vi "test Filters.vi"(8 "error in (no error)":errorcluster, 11 "BM Filters in":refnum<class "BM Filters.lvclass">) -> (0 "error out":errorcluster, 3 "BM Filters out":refnum<class "BM Filters.lvclass">)   [LabVIEW 2016, in "BM Filters.lvclass"]
uses:
  BM Filters.lvclass
  Filters/Filter/Filter.lvclass
  Frames & Messages/TypeDefs/Command Type.ctl
  BCI-1553 API.lvlib
  Filters/TypeDefs/Filter Configuration.ctl
  1553 Component/1553 Component.lvclass
  Bus Monitor/TypeDefs/Bus Monitor Configuration.ctl
  Bus Monitor/Bus Monitor.lvclass
  1553 Board/1553 Board.lvclass
  PPLs/FPGA Interface.lvlibp/FPGA Interface/FPGA Interface.lvclass
  Utilities/FPGA Interface/FPGA Interface.lvclass
  D:/SVN/Products/BCI-1553/Software/Development/2016/RealTime/1553 SubComponent/1553 SubComponent.lvclass
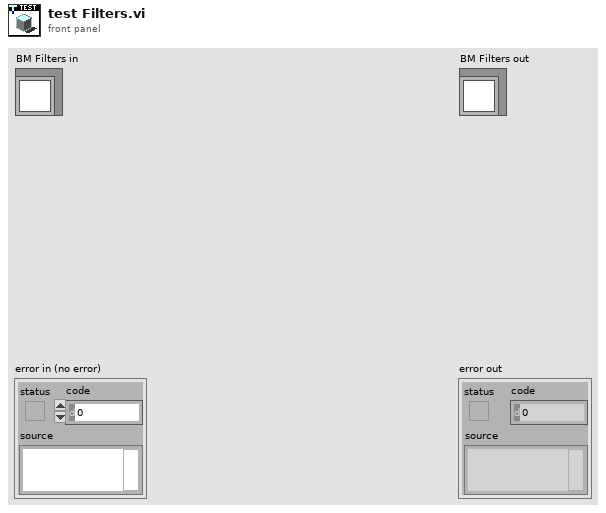
[diagram p1: front panel]
types:
  T1 = typedef "BCI-1553 API.lvlib/Bus Monitor.lvclass/Bus Monitor Configuration.ctl" = cluster{"BM Timeout":u8, "Gap Check":bool, "BM Time Tag Msg Bit Select":u8, "BM Start Record Req":u8, "Cont Record After Inv Word":bool, "Ext Msg Flag Enable":bool, "48-bit Time Tag":bool}
  T2 = typedef "BCI-1553 API.lvlib/Command Type.ctl" = enum16{"Transmit", "Receive"}
  T3 = typedef "BCI-1553 API.lvlib/Filter Configuration.ctl" = cluster{"Filter Type":T2, "Terminal Address (0-30)":u16, "SubAddress (1-30)":u16, "Mode Code":bool, "Broadcast":bool, "RT-RT":bool, "Bus A":bool}
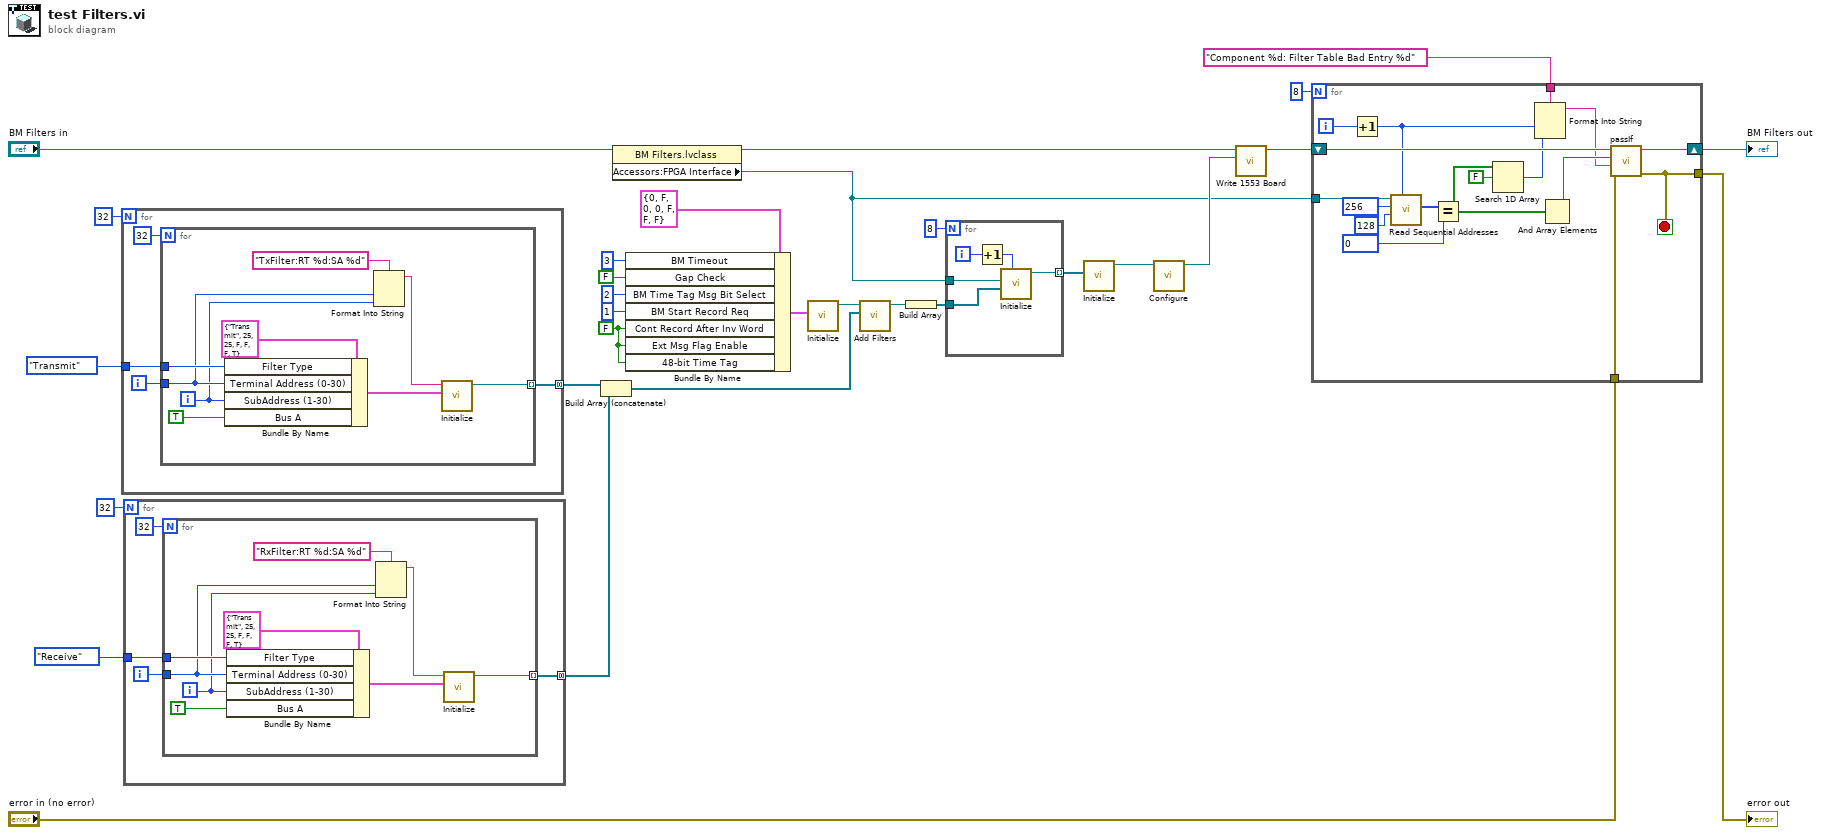
[diagram p0: block diagram]
diagram:
  w19 = FALSE ("Cont Record After Inv Word")
  n1 = for {
    N: 32 -> [_]
    tunnel: Command_Type."Transmit" ("Filter Type") -> [w34]
    tunnel: [w31] -> w26 mode=concatenating
    i -> [w32]
    n2 = for {
      N: 32 -> [_]
      tunnel: w34 -> [w42]
      tunnel: w32 -> [w37]
      tunnel: [w39] -> w31 mode=indexing
      i -> [w36]
      n3 = Bundle By Name(cluster=T3 {"Filter Type"=enum."Transmit", "Terminal Address (0-30)"=25, "SubAddress (1-30)"=25, "Mode Code"=FALSE, "Broadcast"=FALSE, "RT-RT"=FALSE, "Bus A"=TRUE} ("Filter Configuration"), "Filter Type"=w42, "Terminal Address (0-30)"=w37, "SubAddress (1-30)"=w36, "Bus A"=TRUE) -> (w40:T3)
      n4 = Format Into String(format string="TxFilter:RT %d:SA %d", w37, w36) -> (resulting string=w35:string)  [unwired: 2 in, 1 out]
      n5 = call "Initialize.vi"("Filter Configuration"=w40, "ID"=w35) -> ("Filter out"=w39:refnum<class "Filter.lvclass">)  [unwired: 8 in, 1 out]
    }
  }
  n6 = for {
    N: 32 -> [_]
    tunnel: Command_Type."Receive" ("Filter Type") -> [w47]
    tunnel: [w44] -> w25 mode=concatenating
    i -> [w45]
    n7 = for {
      N: 32 -> [_]
      tunnel: w47 -> [w55]
      tunnel: w45 -> [w50]
      tunnel: [w52] -> w44 mode=indexing
      i -> [w49]
      n8 = Bundle By Name(cluster=T3 {"Filter Type"=enum."Transmit", "Terminal Address (0-30)"=25, "SubAddress (1-30)"=25, "Mode Code"=FALSE, "Broadcast"=FALSE, "RT-RT"=FALSE, "Bus A"=TRUE} ("Filter Configuration"), "Filter Type"=w55, "Terminal Address (0-30)"=w50, "SubAddress (1-30)"=w49, "Bus A"=TRUE) -> (w53:T3)
      n9 = Format Into String(format string="RxFilter:RT %d:SA %d", w50, w49) -> (resulting string=w48:string)  [unwired: 2 in, 1 out]
      n10 = call "Initialize.vi"("Filter Configuration"=w53, "ID"=w48) -> ("Filter out"=w52:refnum<class "Filter.lvclass">)  [unwired: 8 in, 1 out]
    }
  }
  n11 = Build Array (concatenate)(w26, w25) -> (w16:refnum<class "Filter.lvclass">[])
  n12 = property class="BM Filters.lvclass"(reference="BM Filters in") -> (reference out=w10:refnum<class "BM Filters.lvclass">, "Accessors:FPGA Interface"=w7:refnum<class "FPGA Interface.lvclass">)  [unwired: 1 in, 1 out]
  n13 = Bundle By Name(cluster=T1 {"BM Timeout"=0, "Gap Check"=FALSE, "BM Time Tag Msg Bit Select"=0, "BM Start Record Req"=0, "Cont Record After Inv Word"=FALSE, "Ext Msg Flag Enable"=FALSE, "48-bit Time Tag"=FALSE} ("Bus Monitor Configuration"), "BM Timeout"=u8 3, "Gap Check"=FALSE, "BM Time Tag Msg Bit Select"=u8 2, "BM Start Record Req"=u8 1, "Cont Record After Inv Word"=w19, "Ext Msg Flag Enable"=w19, "48-bit Time Tag"=w19) -> (w18:T1)
  n14 = call "Initialize.vi"("Bus Monitor Configuration"=w18) -> ("Bus Monitor out"=w17:refnum<class "Bus Monitor.lvclass">)  [unwired: 9 in, 1 out]
  n15 = call-dynamic "Add Filters.vi"("Filters"=w16, "Bus Monitor in"=w17) -> ("Bus Monitor out"=w13:refnum<class "Bus Monitor.lvclass">)  [unwired: 8 in, 1 out]
  n16 = Build Array(w13) -> (w12:refnum<class "Bus Monitor.lvclass">[])
  n17 = for {
    N: 8 -> [_]
    tunnel: w7 -> [w59]
    tunnel: w12 -> [w58]
    tunnel: [w57] -> w11 mode=indexing
    i -> [w61]
    n18 = Increment(x=w61) -> (x+1=w60:i32)
    n19 = call "Initialize.vi"("Component ID (1-8)"=w60, "SubComponents"=w58, "FPGA Interface"=w59) -> ("1553 Component out"=w57:refnum<class "1553 Component.lvclass">)  [unwired: 7 in, 1 out]
  }
  n20 = call "Initialize.vi"("Components"=w11) -> ("1553 Board out"=w9:refnum<class "1553 Board.lvclass">)  [unwired: 9 in, 1 out]
  n21 = call-dynamic "Configure.vi"("1553 Board in"=w9) -> ("1553 Board out"=w8:refnum<class "1553 Board.lvclass">)  [unwired: 9 in, 1 out]
  n22 = call-dynamic "Write 1553 Board.vi"("1553 Board"=w8, "1553 Test in"=w10) -> ("1553 Test out"=w6:refnum<class "BM Filters.lvclass">)  [unwired: 8 in, 1 out]
  n23 = for {
    N: 8 -> [_]
    tunnel: w7 -> [w71]
    shift-right: [w77] -> w1
    shift-left: w6 -> [w78]
    tunnel: [w76] -> w3
    tunnel: "error in (no error)" -> [w75]
    tunnel: "Component %d: Filter Table Bad Entry %d" ("custom report message (\"\")") -> [w69]
    i -> [w74]
    stop <- w76 stop-if-true
    n24 = Increment(x=w74) -> (x+1=w70:i32)
    n25 = call-dynamic "Read Sequential Addresses.vi"("Target IC (1-8)"=w70, "Addresses to Read"=u16 128, "Starting Address"=u16 256, "FPGA Interface in"=w71) -> ("Data"=w68:u16[])  [unwired: 6 in, 1 out]
    n26 = Equal?(x=w68, y=u16 0) -> (x = y?=w64:bool[])
    n27 = Search 1D Array(1D array=w64, element=FALSE) -> (index of element=w62:i32)  [unwired: 1 in]
    n28 = Format Into String(format string=w69, w70, w62) -> (resulting string=w65:string)  [unwired: 2 in, 1 out]
    n29 = And Array Elements(Boolean array=w64) -> (logical AND=w66:bool)
    n30 = call-dynamic "passIf.vi"("error in (no error)"=w75, "message (\"\")"=w65, "pass"=w66, "TestCase in"=w78) -> ("error out"=w76:errorcluster, "TestCase out"=w77:refnum<class "BM Filters.lvclass">)  [unwired: 6 in]
  }
  "error out" <- w3
  "BM Filters out" <- w1
